vi "Config Laser.vi"(0 "Enable laser mode":bool, 5 "Controller ID":T1, 11 "error in (no error)":errorcluster) -> (15 "error out":errorcluster)   [LabVIEW 2024, in "GRBL 1.1.lvlib"]
doc: "Laser-mode enable: Enables laser mode. Consecutive G1/2/3 commands will not halt when spindle speed is changed."
uses:
  GRBL 1.1.lvlib
  Controller ID.ctl
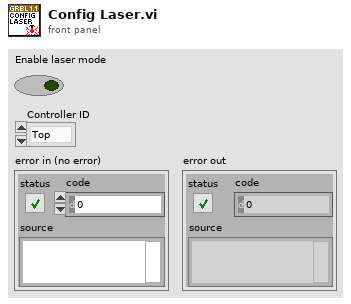
[diagram p1: front panel]
types:
  T1 = typedef "GRBL 1.1.lvlib/Controller ID.ctl" = enum16{"Top", "Bottom"}
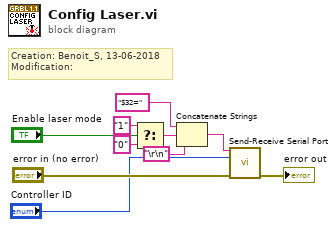
[diagram p0: block diagram]
diagram:
  # "Creation: Benoit_S, 13-06-2018\nModification:"
  n1 = Select(t="1", s="Enable laser mode", f="0") -> (s? t:f=w7:string)
  n2 = Concatenate Strings("$32=", w7, "\r\n") -> (w5:string)
  n3 = call "Send-Receive Serial Port.vi"("Data to write"=w5, 5:"Controller ID", "error in (no error)"="error in (no error)") -> ("error out"=→"error out":errorcluster)  [unwired: 11 in, 1 out]
